vi "SV Append Data.vi"   [LabVIEW 2017]
doc: "Use this VI to buffer data by appending input data to previously buffered data. Set the <B>maximum length</B> to set the buffered array size. The VI functions like a FIFO (First In, First Out) buffer, meaning that the oldest data is overwritten as new elements are added to the buffer. Wire data to the <B>data in</B> input to determine the polymorphic instance to use or manually select the instance."
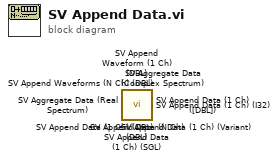
[diagram p0: block diagram]
diagram:
  n1 = call <vilib>:"SV Append Data (N Ch) (DBL).vi"() -> ()  [unwired: 11 in, 1 out]
  n2 = call <vilib>:"SV Aggregate Data (Complex Spectrum).vi"() -> ()  [unwired: 11 in, 1 out]
  n3 = call <vilib>:"SV Aggregate Data (Real Spectrum).vi"() -> ()  [unwired: 11 in, 1 out]
  n4 = call <vilib>:"SV Append Data (1 Ch) ([DBL]).vi"() -> ()  [unwired: 11 in, 1 out]
  n5 = call <vilib>:"SV Append Waveforms (N Ch) (DBL).vi"() -> ()  [unwired: 10 in, 2 out]
  n6 = call <vilib>:"SV Append Waveform (1 Ch) (DBL).vi"() -> ()  [unwired: 10 in, 2 out]
  n7 = call <vilib>:"SV Append Data (1 Ch) (Variant).vi"() -> ()  [unwired: 11 in, 1 out]
  n8 = call <vilib>:"SV Append Data (1 Ch) (SGL).vi"() -> ()  [unwired: 11 in, 1 out]
  n9 = call <vilib>:"SV Append Data (1 Ch) (I32).vi"() -> ()  [unwired: 11 in, 1 out]
  n10 = call <vilib>:"SV Append Data (1 Ch) (DBL).vi"() -> ()  [unwired: 11 in, 1 out]
